vi "Create Accuracy Sort Keys.vi"(8 "error in (no error)":errorcluster, 11 "Accuracy Results":T1[](array[typedef]) {"Accuracy Percent FS" format="%#_3g"}) -> (0 "error out":errorcluster, 3 "Sort Keys":dbl[](array[numeric]))   [LabVIEW 2026, in "Analysis.lvlib"]
uses:
  Analysis.lvlib
  Accuracy Result.ctl
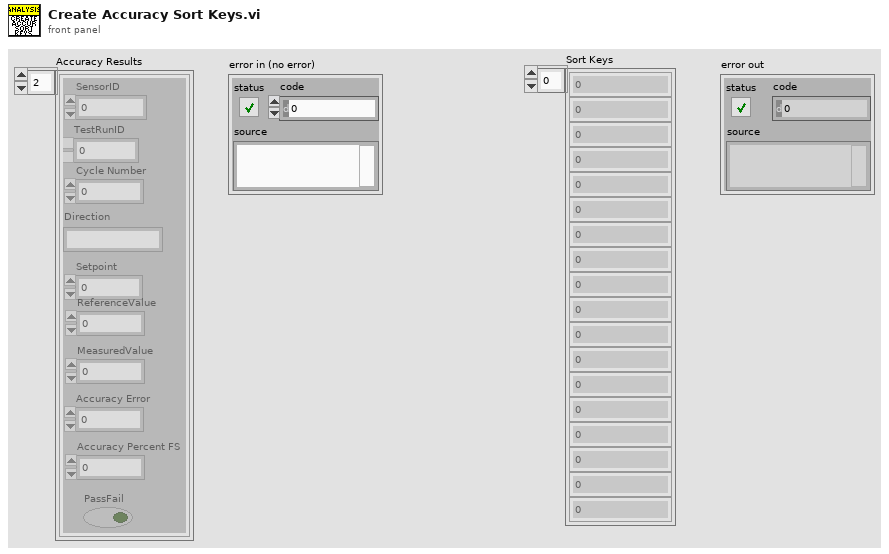
[diagram p1: front panel]
types:
  T1 = typedef "Analysis.lvlib/Accuracy Result.ctl" = cluster{"Setpoint":dbl, "Cycle Number":i32, "SensorID":i32, "TestRunID":i32, "ReferenceValue":dbl, "MeasuredValue":dbl, "Accuracy Percent FS":dbl, "PassFail":bool, "Accuracy Error":dbl, "Direction":string}
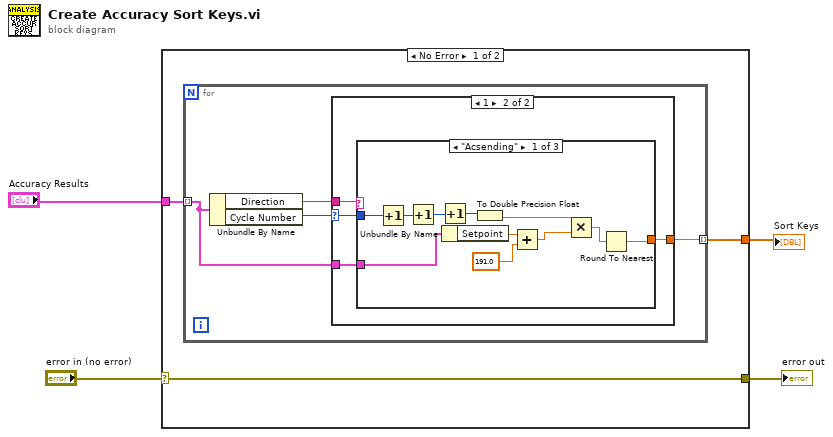
[diagram p0: block diagram]
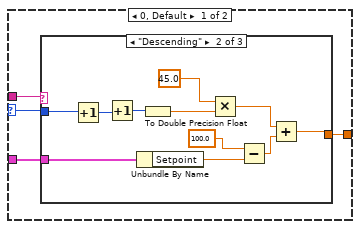
[diagram p2: hidden frame]
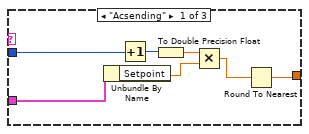
[diagram p3: hidden frame]
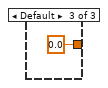
[diagram p4: hidden frame]
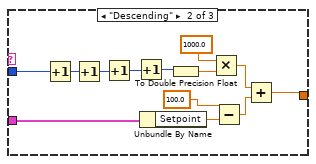
[diagram p5: hidden frame]
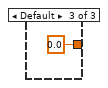
[diagram p6: hidden frame]
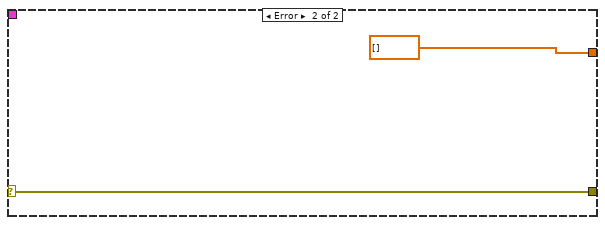
[diagram p7: hidden frame]
diagram:
  n1 = case shown="No Error" "error in (no error)" {
    selector: "error in (no error)" -> [w6 w65]
    tunnel: "Accuracy Results" -> [w7 _]
    tunnel: [w6 w65] -> w3
    tunnel: [w5 dbl[] []] -> w2
    frame No Error {
      n2 = for {
        tunnel: w7 -> [w10] mode=indexing
        tunnel: [w9] -> w5 mode=indexing
        n3 = Unbundle By Name(w10) -> ("Direction"=w11:string, "Cycle Number"=w8:i32)
        n4 = case shown="1" w8 {
          selector: w8 -> [w12 w35]
          tunnel: w11 -> [w15 w38]
          tunnel: w10 -> [w14 w37]
          tunnel: [w13 w36] -> w9
          frame 0, Default {
            n5 = case shown="\"Descending\"" w15 {
              tunnel: w14 -> [w22 w33 _]
              tunnel: [w21 w30 0.0 ("Setpoint")] -> w13
              tunnel: w12 -> [w17 w24 _]
              frame "Acsending" {
                n6 = Unbundle By Name(w22) -> ("Setpoint"=w20:dbl)
                n7 = Increment(x=w17) -> (x+1=w18:i32)
                n8 = To Double Precision Float(number=w18) -> (double precision float=w16:dbl)
                n9 = Multiply(x=w16, y=w20) -> (x*y=w19:dbl)
                n10 = Round To Nearest(number=w19) -> (nearest integer value=w21:dbl)
              }
              frame "Descending" {
                n11 = Increment(x=w24) -> (x+1=w26:i32)
                n12 = Increment(x=w26) -> (x+1=w25:i32)
                n13 = Unbundle By Name(w33) -> ("Setpoint"=w32:dbl)
                n14 = To Double Precision Float(number=w25) -> (double precision float=w23:dbl)
                n15 = Multiply(x=45.0, y=w23) -> (x*y=w27:dbl)
                n16 = Subtract(x=100.0, y=w32) -> (x-y=w31:dbl)
                n17 = Add(x=w27, y=w31) -> (x+y=w30:dbl)
              }
              frame Default {
              }
            }
          }
          frame 1 {
            n18 = case shown="\"Acsending\"" w38 {
              tunnel: w37 -> [w49 w62 _]
              tunnel: [w48 w58 0.0 ("Setpoint")] -> w36
              tunnel: w35 -> [w42 w53 _]
              frame "Acsending" {
                n19 = Increment(x=w42) -> (x+1=w46:i32)
                n20 = Increment(x=w46) -> (x+1=w45:i32)
                n21 = Increment(x=w45) -> (x+1=w44:i32)
                n22 = Unbundle By Name(w49) -> ("Setpoint"=w41:dbl)
                n23 = To Double Precision Float(number=w44) -> (double precision float=w43:dbl)
                n24 = Add(x=w41, y=191.0) -> (x+y=w39:dbl)
                n25 = Multiply(x=w43, y=w39) -> (x*y=w47:dbl)
                n26 = Round To Nearest(number=w47) -> (nearest integer value=w48:dbl)
              }
              frame "Descending" {
                n27 = Increment(x=w53) -> (x+1=w52:i32)
                n28 = Increment(x=w52) -> (x+1=w51:i32)
                n29 = Increment(x=w51) -> (x+1=w55:i32)
                n30 = Increment(x=w55) -> (x+1=w54:i32)
                n31 = Unbundle By Name(w62) -> ("Setpoint"=w60:dbl)
                n32 = To Double Precision Float(number=w54) -> (double precision float=w50:dbl)
                n33 = Multiply(x=1000.0, y=w50) -> (x*y=w57:dbl)
                n34 = Subtract(x=100.0, y=w60) -> (x-y=w59:dbl)
                n35 = Add(x=w57, y=w59) -> (x+y=w58:dbl)
              }
              frame Default {
              }
            }
          }
        }
      }
    }
    frame Error {
    }
  }
  "Sort Keys" <- w2
  "error out" <- w3
